vi "2D DBL Array_Delete Repeating Sells_Column Selection.vi"(1 "Column":i32, 2 "2D DBL Array.In":dbl[][](array[numeric])) -> (6 "2D DBL Array.Out":dbl[][](array[numeric]))   [LabVIEW 2020]
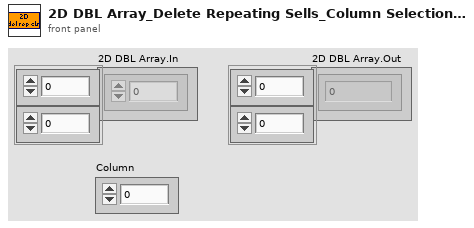
[diagram p1: front panel]
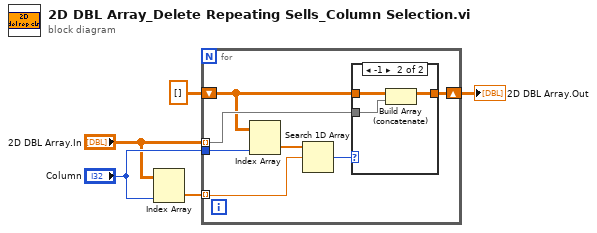
[diagram p0: block diagram]
diagram:
  n1 = Index Array(array="2D DBL Array.In", index (col)="Column") -> (element=w4:dbl[])  [unwired: 1 in]
  n2 = for {
    shift-right: [w11] -> w1
    shift-left: dbl[][] [] ("sorted array") -> [w6]
    tunnel: w4 -> [w8] mode=indexing
    tunnel: "Column" -> [w10]
    tunnel: "2D DBL Array.In" -> [w7] mode=indexing
    n3 = Index Array(array=w6, index (col)=w10) -> (element=w9:dbl[])  [unwired: 1 in]
    n4 = Search 1D Array(1D array=w9, element=w8) -> (index of element=w12:i32)  [unwired: 1 in]
    n5 = case shown="-1" w12 {
      tunnel: w7 -> [_ w14]
      tunnel: [w13 w16] -> w11
      tunnel: w6 -> [w13 w15]
      frame 0, Default {
      }
      frame -1 {
        n6 = Build Array (concatenate)(w15, w14) -> (w16:dbl[][])
      }
    }
  }
  "2D DBL Array.Out" <- w1
